vi "Get Connection List.vi"(8 "error in (no error)":errorcluster, 11 "PIPXI40 Switching in":refnum<class "PIPXI40 GP Switch.lvclass">) -> (0 "error out":errorcluster, 2 "List":variant, 3 "PIPXI40 Switching out":refnum<class "PIPXI40 GP Switch.lvclass">)   [LabVIEW 2020, in "PIPXI40.lvlib" / "PIPXI40 GP Switch.lvclass"]
uses:
  PIPXI40 GP Switch.lvclass
  D:/WSGitHub/RTFWK/Realization/PIPXI40 Base/PIPXI40 Base.lvclass
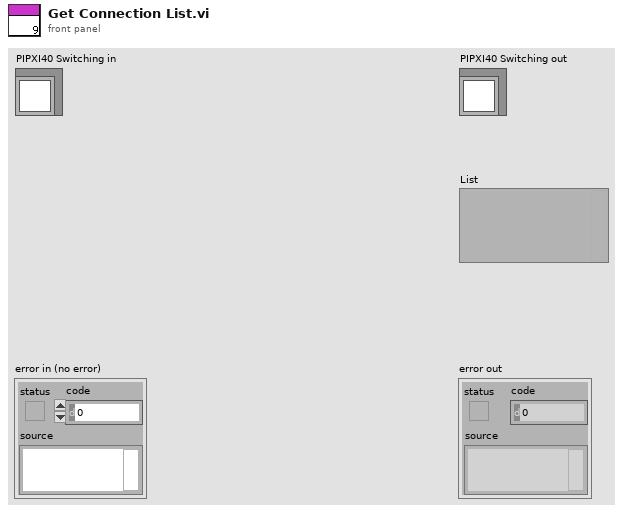
[diagram p1: front panel]
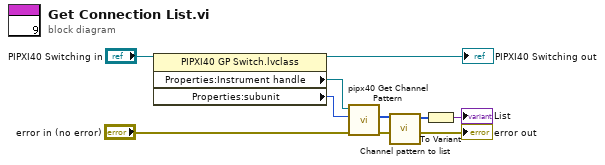
[diagram p0: block diagram]
diagram:
  n1 = property class="PIPXI40 GP Switch.lvclass"(reference="PIPXI40 Switching in") -> (reference out=→"PIPXI40 Switching out":refnum<class "PIPXI40 GP Switch.lvclass">, "Properties:Instrument handle"=w6:refnum<visa-resource-name>, "Properties:subunit"=w5:u32)  [unwired: 1 in, 1 out]
  n2 = call <instrlib>:"pipx40 Get Channel Pattern.vi"("error in (no error)"="error in (no error)", "subunit number"=w5, "instrument handle"=w6) -> ("error out"=→"error out":errorcluster, "pattern"=w3:u32[])  [unwired: 6 in, 1 out]
  n3 = call "Channel pattern to list.vi"("Pattern"=w3) -> ("List"=w2:i32[])  [unwired: 10 in]
  n4 = To Variant(anything=w2) -> (Variant=→"List":variant)
